vi "Invoke Commands.vi"(10 "Command Params":string[][](array[string]), 11 "Function Name":string) -> (0 "Params":u8, 1 "Started":bool, 2 "Unique ID":u16)   [LabVIEW 2017]
uses:
  <vilib>/Rock Robotics/Network Tables/NT Globals.vi
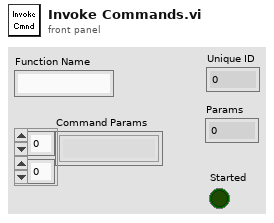
[diagram p1: front panel]
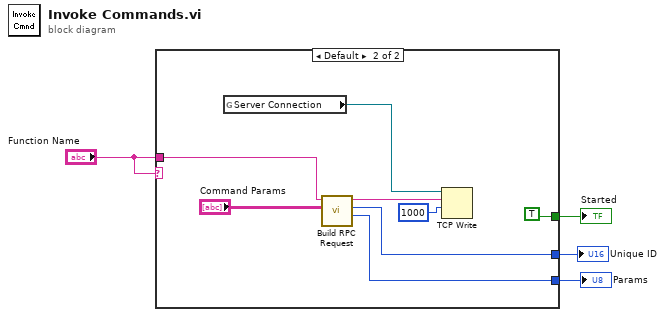
[diagram p0: block diagram]
diagram:
  n1 = case shown="Default" "Function Name" {
    tunnel: "Function Name" -> [_ w8]
    tunnel: [_ w7] -> w3
    tunnel: [_ w6] -> w2
    tunnel: [_ TRUE] -> w1
    frame "" {
    }
    frame Default {
      n2 = global read "NT Globals.vi" "Server Connection"() -> (w10:refnum<k5>)
      n3 = call <vilib>:"Build RPC Request.vi"("Command Params"="Command Params", "VI Name"=w8) -> ("Params"=w6:u8, "Unique ID"=w7:u16, "Command Buffer"=w11:string)  [unwired: 7 in]
      n4 = TCP Write(connection ID=w10, data in=w11, 9:1000 ("timeout ms (25000)")) -> ()  [unwired: 1 in, 3 out]
    }
  }
  "Unique ID" <- w3
  "Params" <- w2
  "Started" <- w1
